vi "ToString.vi"(8 "error in (no error)":errorcluster, 11 "String Starts With in":refnum<class "String Starts With.lvclass">) -> (0 "error out":errorcluster, 2 "String":string, 3 "String Starts With out":refnum<class "String Starts With.lvclass">)   [LabVIEW 2017, in "Transparent Assertions.lvlib" / "Constraints.lvlib" / "String Starts With.lvclass"]
doc: "Returns a string representation of the object."
uses:
  String Starts With.lvclass
  String Starts With.lvclass/String Starts With.ctl
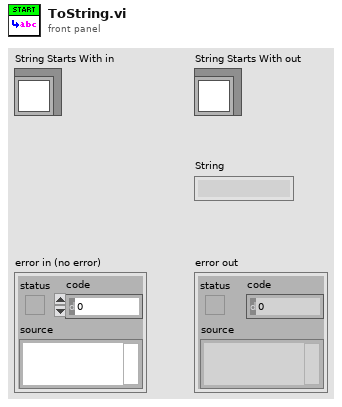
[diagram p1: front panel]
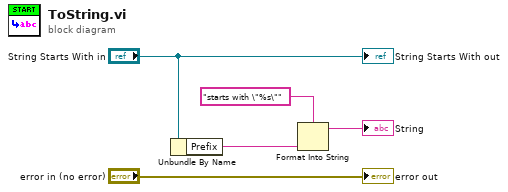
[diagram p0: block diagram]
diagram:
  n1 = Unbundle By Name("String Starts With in") -> ("Prefix"=w1:string)
  n2 = Format Into String(format string="starts with \"%s\"", w1) -> (resulting string=→"String":string)  [unwired: 2 in, 1 out]
  "error out" <- "error in (no error)"
  "String Starts With out" <- "String Starts With in"
